vi "loadControls.vi"(7 "prevName":string caption="default name", 8 "error in (no error)":errorcluster, 9 "Autoload?":bool, 10 "ControlsToLoad":refnum<vi>[](array[refnum]), 11 "ConfigXMLControls":T1) -> (0 "error out":errorcluster, 3 "nameUsed":string)   [LabVIEW 2015]
uses:
  ConfigXMLControl.ctl
  General/CorePluginInfo.ctl
panel:
  # "Loads the selected controls from an XML file. If autoLoad is selected,\nloads the most recently created autosave file"
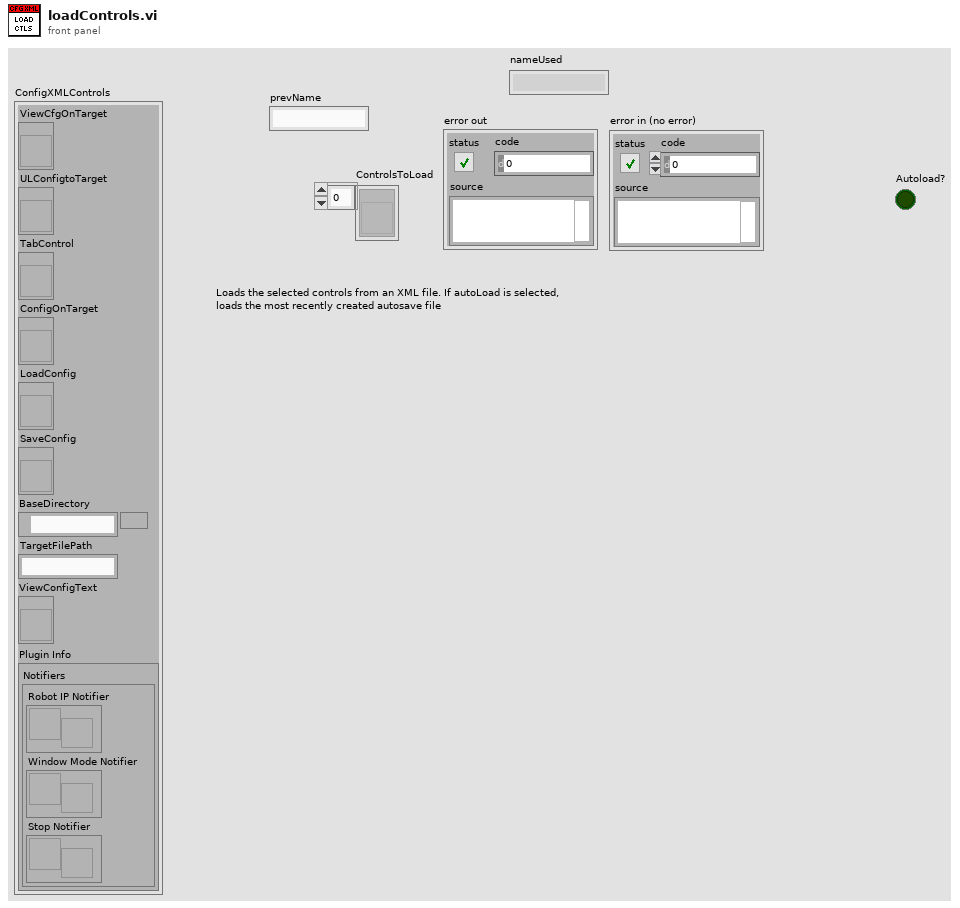
[diagram p1: front panel]
types:
  T1 = typedef "ConfigXMLControl.ctl" = cluster{"ViewCfgOnTarget":refnum<vi>, "ULConfigtoTarget":refnum<vi>, "TabControl":refnum<vi>, "ConfigOnTarget":refnum<vi>, "LoadConfig":refnum<vi>, "SaveConfig":refnum<vi>, "BaseDirectory":path, "TargetFilePath":string, "ViewConfigText":refnum<vi>, "Plugin Info":T2}
  T2 = typedef "CorePluginInfo.ctl" = cluster{"Notifiers":cluster{"Robot IP Notifier":refnum<notifier>, "Window Mode Notifier":refnum<notifier>, "Stop Notifier":refnum<notifier>}}
  T3 = cluster{"appended path":path, "File Created Date (UTC)":timestamp}
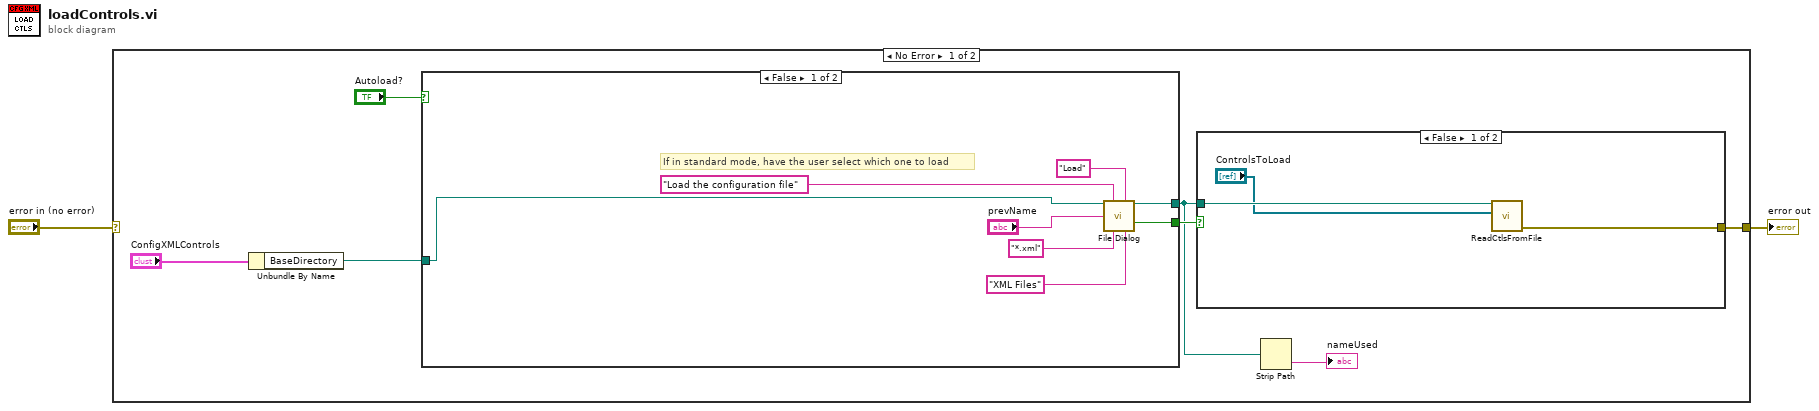
[diagram p0: block diagram]
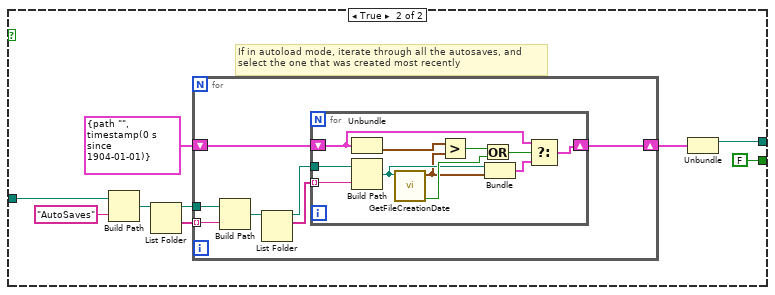
[diagram p3: hidden frame]
diagram:
  n1 = case shown="No Error" "error in (no error)" {
    selector: "error in (no error)" -> [_ w48]
    tunnel: [w5 w48] -> w2
    frame No Error {
      n2 = Unbundle By Name("ConfigXMLControls") -> ("BaseDirectory"=w7:path)
      n3 = case shown="False" "Autoload?" {
        tunnel: w7 -> [w15 w29]
        tunnel: [w13 w22] -> w4
        tunnel: [w14 FALSE ("cancelled")] -> w6
        frame False {
          # "If in standard mode, have the user select which one to load"
          n4 = call "File Dialog"("start path"=w15, "prompt"="Load the configuration file", "button label"="Load", "default name"="prevName", "pattern (all files)"="*.xml", "pattern label"="XML Files") -> ("selected path"=w13:path, "cancelled"=w14:bool)  [unwired: 6 in, 2 out]
        }
        frame True {
          # "If in autoload mode, iterate through all the autosaves, and \nselect the one that was created most recently"
          n5 = Build Path(base path=w29, name or relative path="AutoSaves") -> (appended path=w27:path)
          n6 = List Folder(path=w27) -> (path out=w25:path, folder names=w26:string[])  [unwired: 3 in, 2 out]
          n7 = for {
            tunnel: w26 -> [w34] mode=indexing
            shift-right: [w35] -> w23
            shift-left: cluster{path, timestamp} {path "", timestamp(0 s since 1904-01-01)} -> [w36]
            tunnel: w25 -> [w33]
            n8 = Build Path(base path=w33, name or relative path=w34) -> (appended path=w32:path)
            n9 = List Folder(path=w32) -> (path out=w31:path, filenames=w30:string[])  [unwired: 3 in, 2 out]
            n10 = for {
              shift-right: [w37] -> w35
              shift-left: w36 -> [w38]
              tunnel: w30 -> [w46] mode=indexing
              tunnel: w31 -> [w47]
              n11 = Unbundle(w38) -> (w42:timestamp)  [unwired: 1 out]
              n12 = Build Path(base path=w47, name or relative path=w46) -> (appended path=w41:path)
              n13 = call "GetFileCreationDate.vi"("File Path"=w41) -> ("Error"=w45:bool, "File Created Date (UTC)"=w40:timestamp)  [unwired: 7 in]
              n14 = Greater?(x=w42, y=w40) -> (0:w44:bool)
              n15 = Or(x=w44, y=w45) -> (x .or. y?=w43:bool)
              n16 = Bundle("appended path"=w41, "File Created Date (UTC)"=w40) -> (w39:T3)  [unwired: 1 in]
              n17 = Select(t=w38, s=w43, f=w39) -> (s? t:f=w37:T3)
            }
          }
          n18 = Unbundle(w23) -> (w22:path)  [unwired: 1 out]
        }
      }
      n19 = case shown="False" w6 {
        tunnel: w4 -> [w12 _]
        tunnel: [w10 _] -> w5
        frame False {
          n20 = call "ReadCtlsFromFile.vi"("ControlsToLoad"="ControlsToLoad", "selected path"=w12) -> ("error out"=w10:errorcluster)  [unwired: 9 in]
        }
        frame True {
          # "If true, do not load the controls"
        }
      }
      n21 = Strip Path(path=w4) -> (name=→"nameUsed":string)  [unwired: 1 out]
    }
    frame Error {
    }
  }
  "error out" <- w2
